vi "test_jog.vi"() -> ()   [LabVIEW 2010]
panel:
  out "Array":dbl[][](array[numeric])
  in  "stop":bool
  out "indic":bool
  in  "S":bool
  in  "W":bool
  in  "E":bool
  in  "N":bool
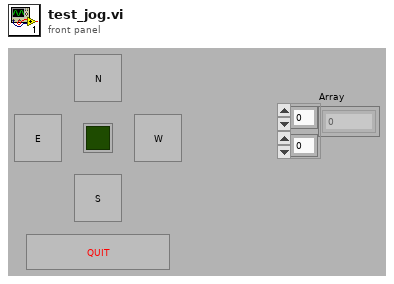
[diagram p1: front panel]
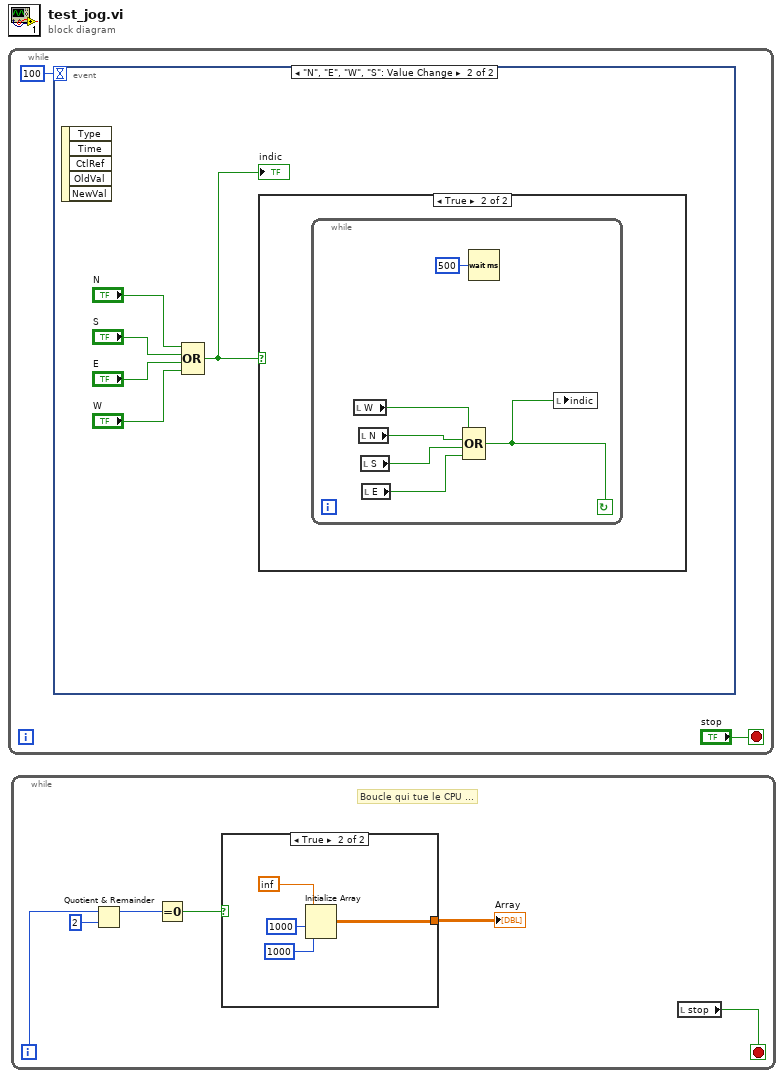
[diagram p0: block diagram]
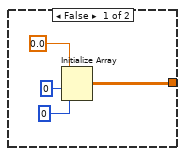
[diagram p2: hidden frame]
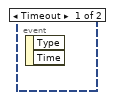
[diagram p3: hidden frame]
diagram:
  n1 = while {
    stop <- "stop" stop-if-true
    n2 = event shown="[1] \"N\", \"E\", \"W\", \"S\": Value Change" {
      selector: _ -> [_ _]
      dyn-events: _ -> [_ _]
      timeout: 100 -> [_ _]
      event Timeout {
        n3 = event-data() -> ()  [unwired: 1 in, 2 out]
      }
      event "N", "E", "W", "S": Value Change {
        n4 = event-data() -> ()  [unwired: 1 in, 5 out]
        n5 = Compound Arithmetic op=OR("N", "S", "E", "W") -> (w3:bool)
        "indic" <- w3
        n6 = case shown="True" w3 {
          frame False {
          }
          frame True {
            n7 = while {
              stop <- w8 continue-if-true
              n8 = local read "W"() -> (w12:bool)
              n9 = local read "N"() -> (w11:bool)
              n10 = local read "S"() -> (w10:bool)
              n11 = local read "E"() -> (w9:bool)
              n12 = Compound Arithmetic op=OR(w12, w11, w10, w9) -> (w8:bool)
              n13 = Wait (ms)(milliseconds to wait=u32 500) -> ()  [unwired: 1 out]
              n14 = local write "indic"(w8) -> ()
            }
          }
        }
      }
    }
  }
  n15 = while {
    i -> [w18]
    stop <- w19 stop-if-true
    # "Boucle qui tue le CPU ..."
    n16 = Quotient & Remainder(x=w18, y=2) -> (x-y*floor(x/y)=w16:i32)  [unwired: 1 out]
    n17 = Equal To 0?(x=w16) -> (x = 0?=w15:bool)
    n18 = case shown="True" w15 {
      tunnel: [w20 w27] -> w14
      frame False {
        n19 = Initialize Array(0.0, 0 ("dimension size"), 0 ("dimension size")) -> (w20:dbl[][])
      }
      frame True {
        n20 = Initialize Array(inf, 1000 ("dimension size"), 1000 ("dimension size")) -> (w27:dbl[][])
      }
    }
    "Array" <- w14
    n21 = local read "stop"() -> (w19:bool)
  }
